vi "Get DBMax.vi"(8 "error in (no error)":errorcluster caption="entrée d'erreur (pas d'erreur)", 11 "Class Spectrum Analyser (Default) en entrée":refnum<class "Class Spectrum Analyser (Default).lvclass">) -> (0 "error out":errorcluster caption="sortie d'erreur", 2 "DBMax":dbl, 3 "Class Spectrum Analyser (Default) en sortie":refnum<class "Class Spectrum Analyser (Default).lvclass">)   [LabVIEW 2020, in "Library Instrument & Equipement.lvlib" / "Library Spectrum Analyser.lvlib" / "Class Spectrum Analyser (Default).lvclass"]
uses:
  Class Spectrum Analyser (Default).lvclass
  Class Spectrum Analyser (Default).lvclass/Class Spectrum Analyser (Default).ctl
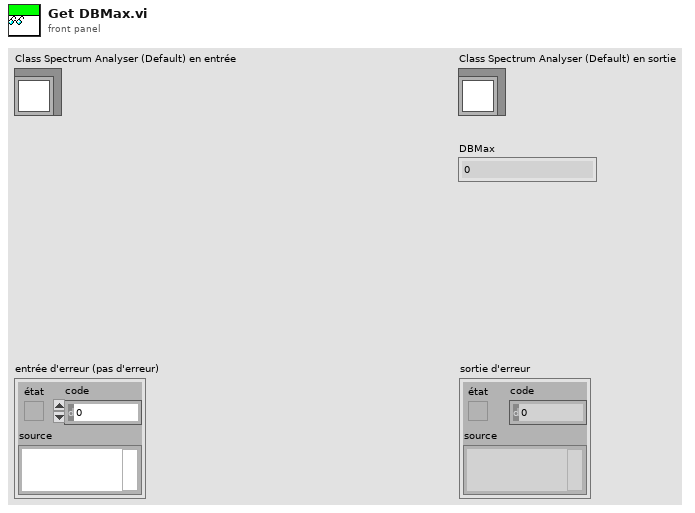
[diagram p1: front panel]
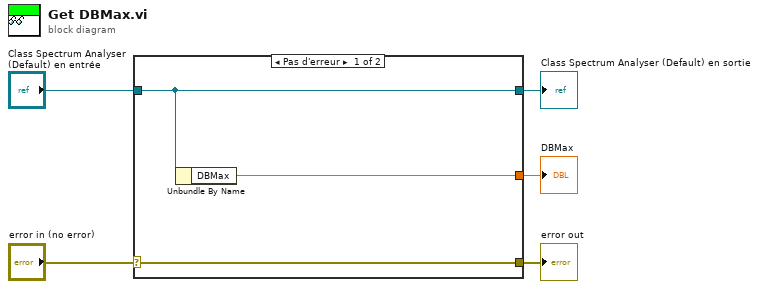
[diagram p0: block diagram]
diagram:
  n1 = case shown="Pas d'erreur" "error in (no error)" {
    selector: "error in (no error)" -> [w8 w9]
    tunnel: [w8 w9] -> w4
    tunnel: [w7 w10] -> w2
    tunnel: "Class Spectrum Analyser (Default) en entrée" -> [w7 w10]
    tunnel: [w6 _] -> w1
    frame No Error {
      n2 = Unbundle By Name(w7) -> ("DBMax"=w6:dbl)
    }
    frame Error {
    }
  }
  "error out" <- w4
  "Class Spectrum Analyser (Default) en sortie" <- w2
  "DBMax" <- w1
